vi "ScanDelay_FTIR_GetSpectrum.vi"(0 "Acquire / Pause? External":refnum<vi>, 1 "% averaged (external)":refnum<vi>, 2 "Binned interferogram (external)":refnum<vi>, 3 "Python refnum in":refnum<k35>, 5 "N delays":i32=30000, 7 "Acquisition cycle (external)":refnum<vi>, 8 "Halt acquisition":bool, 9 "Delay calibration\n          factor":dbl=2.403, 10 "Python error in":errorcluster, 11 "Subtract\ndelay (ps)":dbl=0.45, 12 "Acquisitions per interferogram":i32=2, 13 "Time per acquisition (s)":dbl=1.0, 14 "Sampling rate":dbl=250000.0, 15 "Extract envelope":bool=TRUE) -> (4 "Output spectrum":dbl[][](array[numeric]), 6 "Python error out":errorcluster)   [LabVIEW 2021]
uses:
  ScanDelay/Control_AcquireSpectrum.ctl
  <vilib>/Analysis/Matrix/Numeric/Conversions/Matrix To Array - RM.vi
  <vilib>/Analysis/Matrix/NI_Matrix.lvlib
panel:
  out "Own python session":bool
  out "Refnum errors":errorcluster={"status"=TRUE, "code"=91, "source"="Property Node (arg 1) in GetSpectrum.vi->ScanDelay_DAQ_Fourier_test.vi\n<APPEND>\nProperty Name: <b>Value</b>"}
  out "Spectrum (amplitude)":cluster{dbl[], dbl[]}[](graph)
  out "Spectrum (phase)":cluster{dbl[], dbl[]}(graph)
  out "Interferogram (binned)":cluster{dbl, dbl}[](graph)
  in  "Pause acquisition":bool
  out "% averaged":dbl=100.0
  out "Acquisition cycle":dbl[][](graph)
  out "Python module path":path=path "C:/Users/mnopl/Desktop/Software/LabVIEW/ScanDelay/scandelay.py"
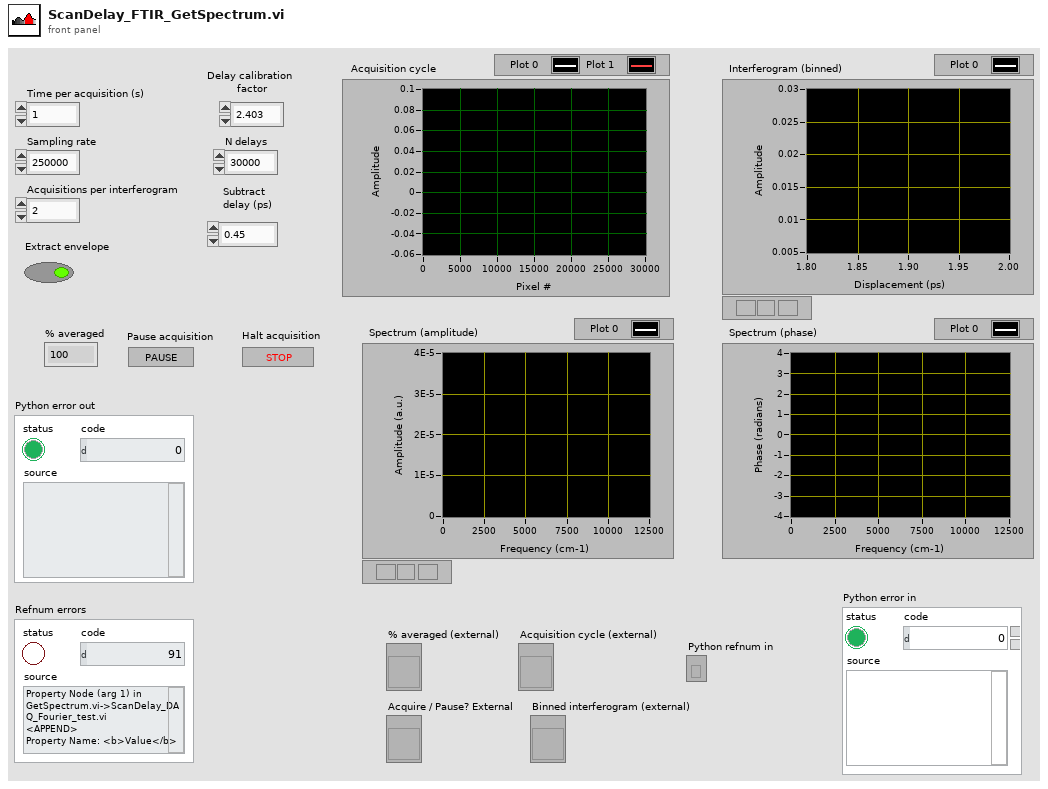
[diagram p1: front panel]
types:
  T1 = typedef "Control_AcquireSpectrum.ctl" = enum16{"Acquire Interferogram", "Bin Interferogram", "Compute Spectrum", "Done"}
  T2 = typedef "NI_Matrix.lvlib/RealMatrix.ctl" = dbl[][]
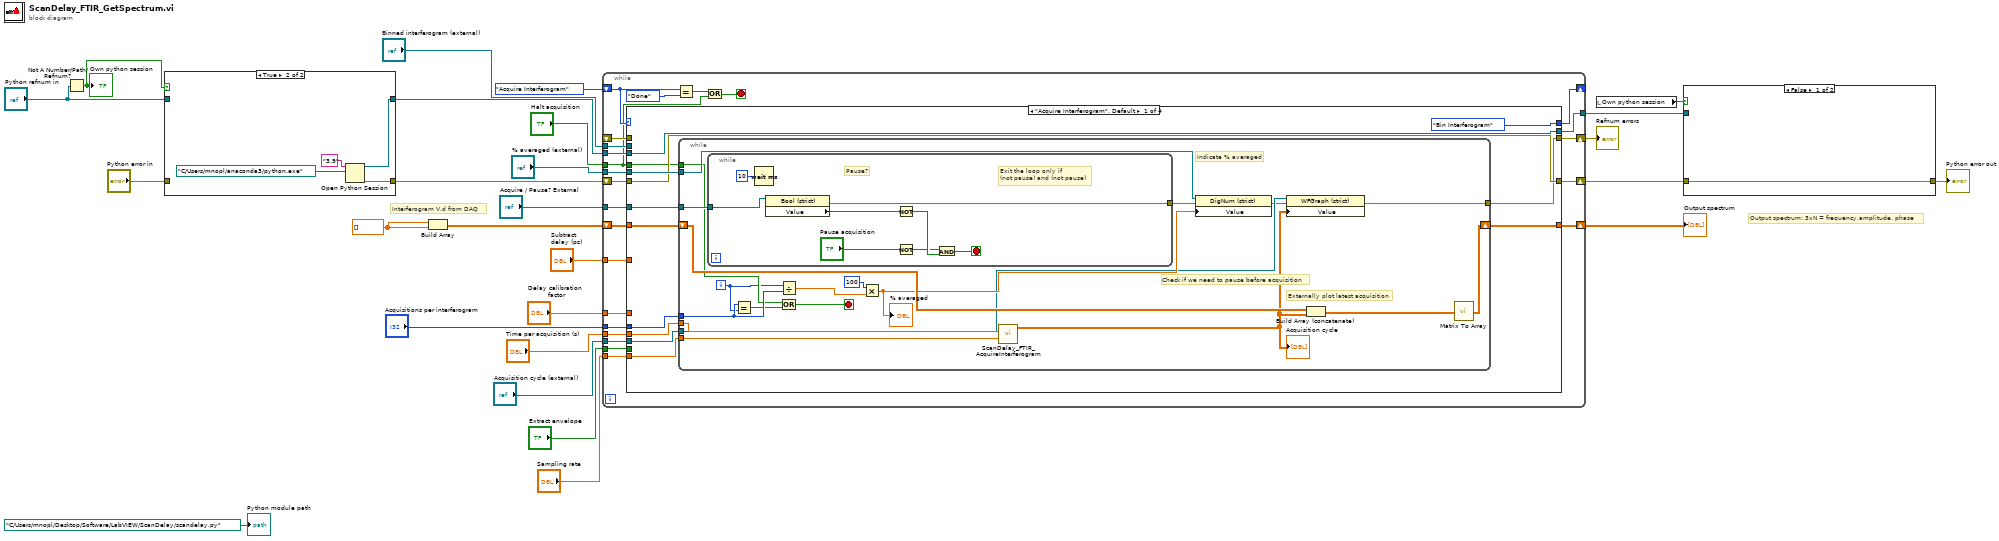
[diagram p0: block diagram]
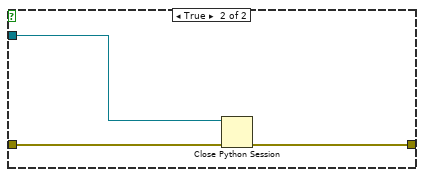
[diagram p2: hidden frame]
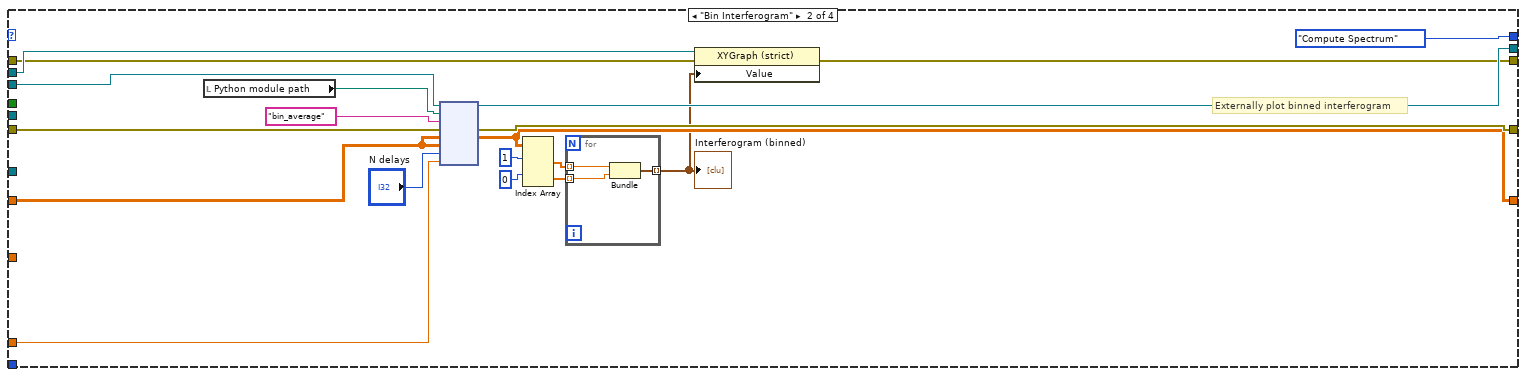
[diagram p4: hidden frame]
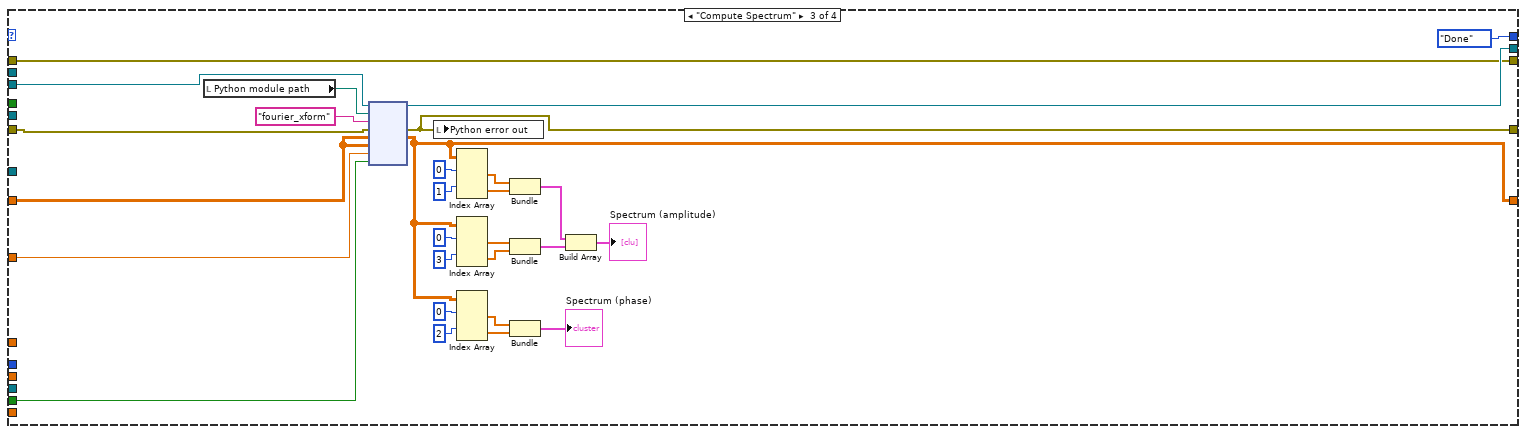
[diagram p5: hidden frame]
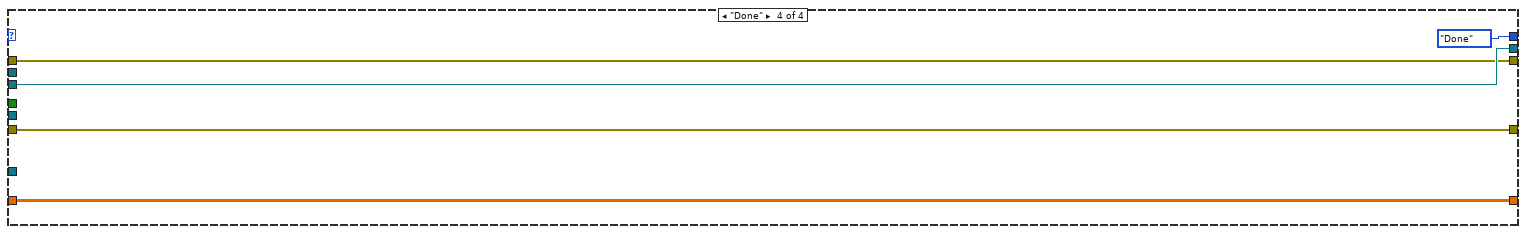
[diagram p6: hidden frame]
diagram:
  w13 = dbl[] []
  # "Output spectrum: 3xN = frequency,amplitude, phase"
  # "Interferogram V,d from DAQ"
  n1 = Not A Number/Path/Refnum?(number/path/refnum="Python refnum in") -> (NaN/Path/Refnum?=w2:bool)
  "Own python session" <- w2
  n2 = case shown="True" w2 {
    tunnel: [w28 w30] -> w6
    tunnel: [w27 w29] -> w5
    tunnel: "Python refnum in" -> [w28 _]
    tunnel: "Python error in" -> [w27 _]
    frame False {
    }
    frame True {
      n3 = Open Python Session(python version="3.9", python path=path "C:/Users/mnopl/anaconda3/python.exe") -> (session out=w30:refnum<k35>, error out=w29:errorcluster)  [unwired: 1 in]
    }
  }
  n4 = Build Array(w13, w13) -> (w12:dbl[][])
  n5 = while {
    shift-right: [w56] -> w11
    shift-left: w12 -> [w55]
    tunnel: w6 -> [w54]
    tunnel: "Acquisition cycle (external)" -> [w52]
    tunnel: "Sampling rate" -> [w51]
    tunnel: "Time per acquisition (s)" -> [w50]
    tunnel: "Delay calibration\n          factor" -> [w49]
    tunnel: "% averaged (external)" -> [w48]
    tunnel: "Acquire / Pause? External" -> [w47]
    tunnel: "Acquisitions per interferogram" -> [w46]
    shift-right: [w45] -> _
    shift-left: Control_AcquireSpectrum."Acquire Interferogram" -> [w43]
    tunnel: "Subtract\ndelay (ps)" -> [w44]
    tunnel: "Halt acquisition" -> [w33]
    tunnel: [w39] -> w15
    shift-right: [w38] -> w10
    shift-left: w5 -> [w53]
    tunnel: "Extract envelope" -> [w37]
    shift-right: [w36] -> w8
    shift-left: _ -> [w35]
    tunnel: "Binned interferogram (external)" -> [w34]
    stop <- w40 stop-if-true
    n6 = case shown="\"Acquire Interferogram\", Default" w43 {
      tunnel: [w69 w101 w126 w152] -> w56
      tunnel: w55 -> [w68 w114 w146 w152]
      tunnel: w54 -> [w61 w113 w145 w150]
      tunnel: w53 -> [w60 w112 w142 w151]
      tunnel: w52 -> [w67 _ _ _]
      tunnel: w51 -> [w66 _ _ _]
      tunnel: w50 -> [w65 _ _ _]
      tunnel: w49 -> [_ w111 _ _]
      tunnel: w48 -> [w64 _ _ _]
      tunnel: w47 -> [w63 _ _ _]
      tunnel: w46 -> [w58 _ _ _]
      tunnel: [w61 w110 w144 w150] -> w39
      tunnel: [Control_AcquireSpectrum."Bin Interferogram" Control_AcquireSpectrum."Compute Spectrum" Control_AcquireSpectrum."Done" Control_AcquireSpectrum."Done"] -> w45
      tunnel: w44 -> [_ _ w141 _]
      tunnel: [w60 w105 w120 w151] -> w38
      tunnel: w37 -> [_ _ w131 _]
      tunnel: [w59 w102 w121 w148] -> w36
      tunnel: w35 -> [_ w103 w121 w148]
      tunnel: w34 -> [_ w104 _ _]
      tunnel: w33 -> [w57 _ _ _]
      frame "Acquire Interferogram", Default {
        n7 = while {
          shift-right: [w88] -> w69
          shift-left: w68 -> [w87]
          tunnel: w67 -> [w78]
          tunnel: w66 -> [w84]
          tunnel: w65 -> [w83]
          tunnel: w64 -> [w82]
          tunnel: w63 -> [w81]
          tunnel: [w75] -> w59
          tunnel: w58 -> [w74]
          tunnel: w57 -> [w71]
          i -> [w70]
          stop <- w72 stop-if-true
          # "Externally plot latest acquisition"
          # "Indicate % averaged"
          # "Check if we need to pause before acquisition"
          n8 = while {
            tunnel: w81 -> [w96]
            tunnel: [w95] -> w76
            stop <- w90 stop-if-true
            # "Exit the loop only if\n(not pause) and (not pause)"
            # "Pause?"
            n9 = Wait (ms)(milliseconds to wait=10) -> ()  [unwired: 1 out]
            n10 = property on="Property Node" class="Bool (strict)"(reference=w96) -> (error out=w95:errorcluster, "Value"=w93:bool)  [unwired: 1 in, 1 out]
            n11 = Not(x=w93) -> (.not. x?=w92:bool)
            n12 = Not(x="Pause acquisition") -> (.not. x?=w91:bool)
            n13 = And(x=w91, y=w92) -> (x .and. y?=w90:bool)
          }
          n14 = Equal?(x=w74, y=w70) -> (x = y?=w73:bool)
          n15 = Divide(x=w70, y=w74) -> (x/y=w86:dbl)
          n16 = Or(x=w71, y=w73) -> (x .or. y?=w72:bool)
          n17 = Multiply(x=100, y=w86) -> (x*y=w80:dbl)
          "% averaged" <- w80
          n18 = call "ScanDelay_FTIR_AcquireInterferogram.vi"("Sampling rate"=w84, "Time per acquisiton (s)"=w83) -> ("Output V-d array"=w79:dbl[][])  [unwired: 9 in]
          "Acquisition cycle" <- w79
          n19 = property on="Property Node" class="DigNum (strict)"(reference=w82, error in=w76, "Value"=w80) -> (error out=w77:errorcluster)  [unwired: 1 out]
          n20 = property on="Property Node" class="WFGraph (strict)"(reference=w78, error in=w77, "Value"=w79) -> (error out=w75:errorcluster)  [unwired: 1 out]
          n21 = Build Array (concatenate)(w87, w79) -> (w89:T2)
          n22 = call-poly <vilib>:"Matrix To Array.vi"("Real Matrix"=w89) -> ("Real 2D Array"=w88:dbl[][])
        }
      }
      frame "Bin Interferogram" {
        # "Externally plot binned interferogram"
        n23 = local read "Python module path"() -> (w109:path)
        n24 = node(w113, w109, "bin_average", w112, w114, w114, "N delays", w111) -> (w110:refnum<k35>, w105:errorcluster, w101:dbl[][])  [unwired: 3 in, 2 out]
        n25 = Index Array(array=w101, index (row) #1=1, index (row) #2=0) -> (element #1=w99:dbl[], element #2=w100:dbl[])  [unwired: 2 in]
        n26 = for {
          tunnel: w100 -> [w118] mode=indexing
          tunnel: w99 -> [w119] mode=indexing
          tunnel: [w117] -> w98 mode=indexing
          n27 = Bundle(w119, w118) -> (w117:cluster{dbl, dbl})  [unwired: 1 in]
        }
        "Interferogram (binned)" <- w98
        n28 = property on="Property Node" class="XYGraph (strict)"(reference=w104, error in=w103, "Value"=w98) -> (error out=w102:errorcluster)  [unwired: 1 out]
      }
      frame "Compute Spectrum" {
        n29 = local read "Python module path"() -> (w143:path)
        n30 = node(w145, w143, "fourier_xform", w142, w146, w146, w141, w131) -> (w144:refnum<k35>, w120:errorcluster, w126:dbl[][])  [unwired: 3 in, 2 out]
        n31 = local write "Python error out"(w120) -> ()
        n32 = Index Array(array=w126, index (row) #1=0, index (row) #2=1) -> (element #1=w137:dbl[], element #2=w136:dbl[])  [unwired: 2 in]
        n33 = Index Array(array=w126, index (row) #1=0, index (row) #2=3) -> (element #1=w132:dbl[], element #2=w133:dbl[])  [unwired: 2 in]
        n34 = Index Array(array=w126, index (row) #1=0, index (row) #2=2) -> (element #1=w127:dbl[], element #2=w128:dbl[])  [unwired: 2 in]
        n35 = Bundle(w137, w136) -> (w124:cluster{dbl[], dbl[]})  [unwired: 1 in]
        n36 = Bundle(w132, w133) -> (w123:cluster{dbl[], dbl[]})  [unwired: 1 in]
        n37 = Bundle(w127, w128) -> (→"Spectrum (phase)":cluster{dbl[], dbl[]})  [unwired: 1 in]
        n38 = Build Array(w124, w123) -> (→"Spectrum (amplitude)":cluster{dbl[], dbl[]}[])
      }
      frame "Done" {
      }
    }
    n39 = Equal?(x=w43, y=Control_AcquireSpectrum."Done") -> (x = y?=w41:bool)
    n40 = Or(x=w41, y=w33) -> (x .or. y?=w40:bool)
  }
  "Output spectrum" <- w11
  "Refnum errors" <- w8
  n41 = local read "Own python session"() -> (w1:bool)
  n42 = case shown="False" w1 {
    tunnel: [w153 w156] -> w16
    tunnel: w15 -> [_ w155]
    tunnel: w10 -> [w153 w154]
    frame False {
    }
    frame True {
      n43 = Close Python Session(session in=w155, error in=w154) -> (11:w156:errorcluster)
    }
  }
  "Python error out" <- w16
  "Python module path" <- path "C:/Users/mnopl/Desktop/Software/LabVIEW/ScanDelay/scandelay.py"
